vi "svfa_Locate Three Fingers (magnitude).vi"(2 "spectrum includes end points?":bool, 3 "criterion":T7={"Single/Multiple"=enum."Multiple Peaks", "Threshold"=0.0, "advanced search"={"approx freq. (optional)"=-1.0, "search (+/- % of Fsampl.)"=5.0}} {"advanced search"."search (+/- % of Fsampl.)" format="%0.2p"; "advanced search"."approx freq. (optional)" format="%0.2p"; "Threshold" format="%.2f"}, 4 "spectrum info":T1={"channel name"="", "description"="", "x-axis units"=0, "spectral info"={"spectrum type"=enum."Power [Magnitude^2]", "linear/dB"=enum."linear", "window"=0, "window size"=0, "FFT size"=0}, "engineering units"=0, "custom label"="", "dB reference [EU]"=0.0, "peak units"=enum."rms", "weighting filter"=0, "spectral density?"=FALSE, "unit label"="", "spectrum skewed?"=FALSE, "complimentary spectrum units"=enum."none"} {"x-axis units" items=["Time (s)"=0, "Frequency-CB (Hz)"=1, "Frequency-CPB (Hz)"=1248, "Frequency-Arbitrary (Hz)"=2357, "Quefrency (s)"=2, "Revolutions (rev)"=3, "Order"=4, "Speed (RPM)"=11, "Speed (rad/s)"=21, "Index"=65535]; "weighting filter" items=["Linear", "A-weighting", "B-weighting", "C-weighting", "ITU-R 468-4", "Dolby", "CCITT", "C-message", "Wb", "Wc", "Wd", "We", "Wf", "Wh", "Wj", "Wk", "Wm", "AES17 20 kHz lowpass", "AES17 40 kHz lowpass", "AES17 20 kHz highpass", "AES17 40 kHz highpass"]; "dB reference [EU]" format="%.2f"; "engineering units" items=["custom..."=0, "V"=1, "A"=21, "C"=30, "pC"=31, "s"=32, "-"=29, "Pa"=2, "N"=20, "g"=3, "m/s^2"=4, "m/s"=5, "m"=6, "mm/s"=12, "mm"=13, "micron/s"=14, "micron"=15, "in/s^2"=7, "in/s"=8, "in"=9, "mil/s"=10, "mil"=11, "rad/s^2"=16, "rad/s"=17, "rad"=18, "deg/s^2"=26, "deg/s"=27, "deg"=28, "RPM"=22, "cycle/s^2"=23, "Hz"=24, "cycle"=25, "strain"=19]; "spectral info"."window" items=["None "=0, "Hanning"=1, "Hamming"=2, "Blackman-Harris"=3, "Exact Blackman"=4, "Blackman"=5, "Flat Top"=6, "4 Term B-Harris "=7, "7 Term B-Harris"=8, "Low Sidelobe"=9, "Force - Exponential"=10, "Gaussian"=62]}, 5 "spectrum":cluster{"f0":dbl, "df":dbl, "magnitude":dbl[]} {"magnitude" format="%.2f"; "df" format="%.2f"; "f0" format="%.2f"}) -> (0 "number of tones":i32, 1 "three fingers (frequency normalized)":cluster{"f0":dbl, "df":dbl, "spectrum":dbl[]}[](array[cluster]) {"spectrum" format="%.2f"; "df" format="%.2e"; "f0" format="%.2e"})   [LabVIEW 2017]
uses:
  <vilib>/addons/_NISVFA/_Shared subVIs/Controls/svc_Spectrum Info.ctl
  <vilib>/addons/_NISVFA/_Shared subVIs/Controls/svc_X-Axis Units.ctl
  <vilib>/addons/_NISVFA/_Shared subVIs/Controls/svc_Spectrum Type.ctl
  <vilib>/addons/_NISVFA/_Shared subVIs/Controls/svc_Engineering Units Text Ring.ctl
  <vilib>/addons/_NISVFA/_Shared subVIs/Controls/svc_Weighting Filter Text Ring.ctl
  <vilib>/addons/_NISVFA/_Shared subVIs/Controls/svc_Complimentary Spectrum Units.ctl
  <vilib>/addons/_NISVFA/_Spectrum Processing/SVFA Get Spectrum Subset (1 Ch).vi
  <vilib>/addons/_NISVFA/_Shared subVIs/Common/svc_Spectrum Units.vi
  <vilib>/addons/_NISVFA/_Shared subVIs/Common/svc_Build Unit Label for Frequency Range.vi
  <vilib>/addons/_NISVFA/_Shared subVIs/Common/svc_Convert Frequency to Frequency String.vi
  <vilib>/addons/_NISVFA/_Shared subVIs/Common/svc_Caller VI Returned in Error Source.vi
  <vilib>/addons/_NISVFA/_Shared subVIs/Common/svc_Check Frequency Range in Spectrum.vi
  <vilib>/addons/_NISVFA/_Shared subVIs/Common/svc_Get Weighting Enum and Labels.vi
  <vilib>/addons/_NISVFA/_Shared subVIs/Common/svc_Unit Label Lexical Class.vi
  <vilib>/addons/_NISVFA/_Shared subVIs/Common/svc_Engineering Units to Unit Label.vi
  <vilib>/addons/_NISVFA/_Shared subVIs/Common/svc_Format Value (DBL).vi
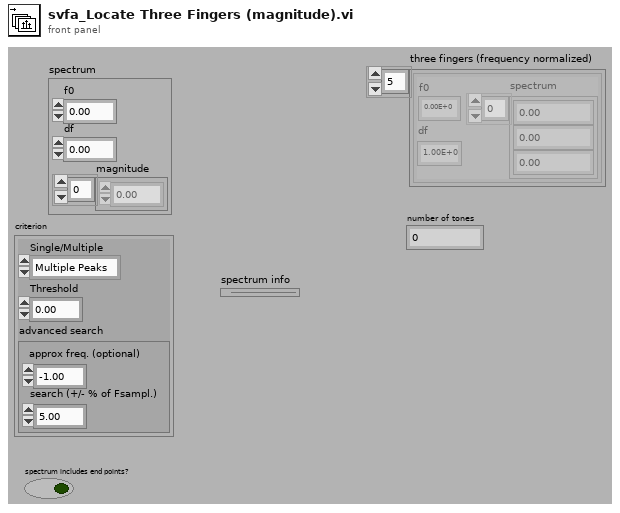
[diagram p1: front panel]
types:
  T1 = typedef "svc_Spectrum Info.ctl" = cluster{"channel name":string, "description":string, "x-axis units":T2, "spectral info":cluster{"spectrum type":T3, "linear/dB":enum16{"linear", "dB"}, "window":u16, "window size":i32, "FFT size":i32}, "engineering units":T4, "custom label":string, "dB reference [EU]":dbl, "peak units":enum16{"rms", "peak", "peak-peak"}, "weighting filter":T5, "spectral density?":bool, "unit label":string, "spectrum skewed?":bool, "complimentary spectrum units":T6}
  T2 = typedef "svc_X-Axis Units.ctl" = u16
  T3 = typedef "svc_Spectrum Type.ctl" = enum16{"FFT Spectrum [complex]", "Amplitude [Magnitude]", "Power [Magnitude^2]", "Cross Spectrum [complex]", "Frequency Response [Complex]"}
  T4 = typedef "svc_Engineering Units Text Ring.ctl" = u16
  T5 = typedef "svc_Weighting Filter Text Ring.ctl" = u16
  T6 = typedef "svc_Complimentary Spectrum Units.ctl" = enum16{"none", "radians", "degrees", "cycles", "imaginary"}
  T7 = cluster{"Single/Multiple":enum16{"Multiple Peaks", "Single Max Peak"}, "Threshold":dbl, "advanced search":cluster{"approx freq. (optional)":dbl, "search (+/- % of Fsampl.)":dbl}}
  T8 = cluster{"start frequency":dbl, "stop frequency":dbl}
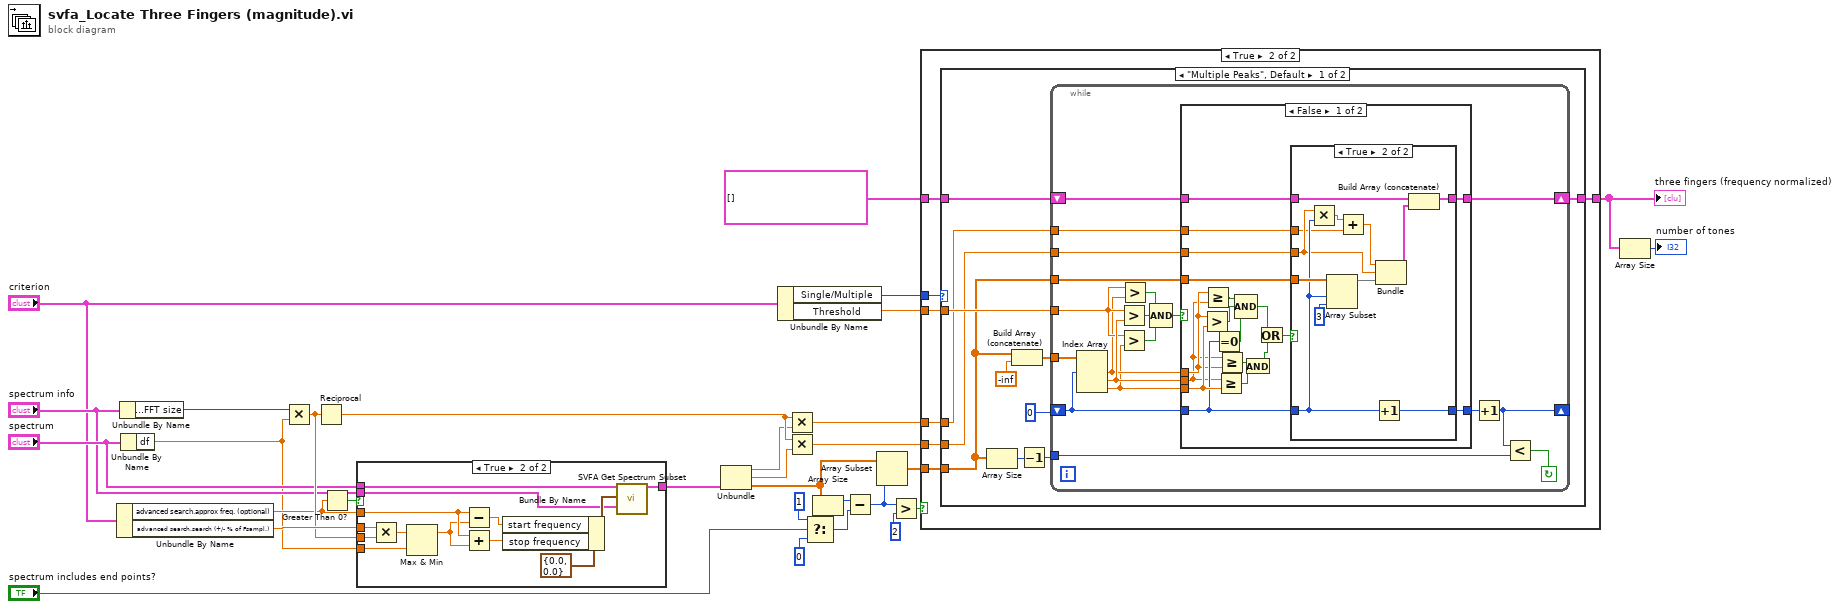
[diagram p0: block diagram]
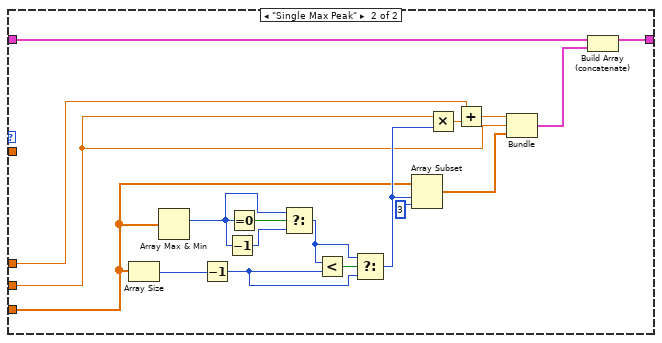
[diagram p6: hidden frame]
diagram:
  n1 = Unbundle By Name("criterion") -> ("advanced search.approx freq. (optional)"=w13:dbl, "advanced search.search (+/- % of Fsampl.)"=w15:dbl)
  n2 = Unbundle By Name("spectrum info") -> ("spectral info.FFT size"=w8:i32)
  n3 = Unbundle By Name("spectrum") -> ("df"=w4:dbl)
  n4 = Multiply(x=w8, y=w4) -> (x*y=w14:dbl)
  n5 = Reciprocal(x=w14) -> (1/x=w16:dbl)
  n6 = Greater Than 0?(x=w13) -> (x > 0?=w12:bool)
  n7 = case shown="True" w12 {
    tunnel: [w31 w34] -> w1
    tunnel: w15 -> [_ w43]
    tunnel: w14 -> [_ w42]
    tunnel: w13 -> [_ w41]
    tunnel: "spectrum" -> [w31 w39]
    tunnel: w4 -> [_ w37]
    tunnel: "spectrum info" -> [_ w33]
    frame False {
    }
    frame True {
      n8 = Multiply(x=w43, y=w42) -> (x*y=w36:dbl)
      n9 = Max & Min(x=w36, y=w37) -> (max(x,y)=w35:dbl)  [unwired: 1 out]
      n10 = Subtract(x=w41, y=w35) -> (x-y=w32:dbl)
      n11 = Add(x=w41, y=w35) -> (x+y=w40:dbl)
      n12 = Bundle By Name(cluster=T8 {"start frequency"=0.0, "stop frequency"=0.0} ("frequency range"), "start frequency"=w32, "stop frequency"=w40) -> (w38:T8)
      n13 = call-poly <vilib>:"SVFA Get Spectrum Subset.vi"("spectrum"=w39, "range"=w38, "spectrum info"=w33) -> ("spectrum subset"=w34:cluster{"x0":dbl, "dx":dbl, "magnitude":dbl[]})  [unwired: 11 in, 5 out]
    }
  }
  n14 = Unbundle(w1) -> ("x0"=w3:dbl, "dx"=w2:dbl, "magnitude"=w5:dbl[])
  n15 = Unbundle By Name("criterion") -> ("Single/Multiple"=w26:enum16{"Multiple Peaks", "Single Max Peak"}, "Threshold"=w27:dbl)
  n16 = Multiply(x=w16, y=w3) -> (x*y=w11:dbl)
  n17 = Multiply(x=w16, y=w2) -> (x*y=w10:dbl)
  n18 = Select(t=1, s="spectrum includes end points?", f=0) -> (s? t:f=w22:i32)
  n19 = Array Size(array=w5) -> (size(s)=w23:i32)
  n20 = Subtract(x=w23, y=w22) -> (x-y=w17:i32)
  n21 = Array Subset(array=w5, length=w17) -> (w18:dbl[])  [unwired: 1 in]
  n22 = Greater?(x=w17, y=2) -> (0:w29:bool)
  n23 = case shown="True" w29 {
    tunnel: w27 -> [_ w52]
    tunnel: w11 -> [_ w51]
    tunnel: w10 -> [_ w50]
    tunnel: [w45 w49] -> w25
    tunnel: w18 -> [_ w48]
    tunnel: cluster{"f0":dbl, "df":dbl, "spectrum":dbl[]}[] [] ("three fingers") -> [w45 w47]
    tunnel: w26 -> [_ w46]
    frame False {
    }
    frame True {
      n24 = case shown="\"Multiple Peaks\", Default" w46 {
        tunnel: w52 -> [w60 _]
        tunnel: w51 -> [w59 w124]
        tunnel: w50 -> [w58 w122]
        tunnel: [w57 w118] -> w49
        tunnel: w48 -> [w53 w117]
        tunnel: w47 -> [w54 w120]
        frame "Multiple Peaks", Default {
          n25 = Array Size(array=w53) -> (size(s)=w56:i32)
          n26 = Build Array (concatenate)(w53, -inf ("df")) -> (w62:dbl[])
          n27 = Decrement(x=w56) -> (x-1=w55:i32)
          n28 = while {
            tunnel: w55 -> [w71]
            tunnel: w58 -> [w75]
            tunnel: w59 -> [w76]
            tunnel: w53 -> [w77]
            shift-left: w54 -> [w78]
            shift-right: [w74] -> w57
            tunnel: w60 -> [w69]
            shift-left: 0 -> [w80]
            shift-right: [w72] -> _
            tunnel: w62 -> [w82]
            stop <- w73 continue-if-true
            n29 = Index Array(array=w82, index #1=w80) -> (element #1=w68:dbl, element #2=w70:dbl, element #3=w67:dbl)  [unwired: 2 in]
            n30 = Greater?(x=w69, y=w70) -> (0:w81:bool)
            n31 = Greater?(x=w69, y=w67) -> (0:w64:bool)
            n32 = Greater?(x=w69, y=w68) -> (0:w65:bool)
            n33 = Compound Arithmetic op=AND(w65, w81, w64) -> (w66:bool)
            n34 = case shown="False" w66 {
              tunnel: [w98 w116] -> w79
              tunnel: w80 -> [w88 w116]
              tunnel: w67 -> [w92 _]
              tunnel: w68 -> [w84 _]
              tunnel: w78 -> [w97 w115]
              tunnel: w77 -> [w96 _]
              tunnel: w76 -> [w95 _]
              tunnel: w75 -> [w94 _]
              tunnel: [w93 w115] -> w74
              tunnel: w70 -> [w83 _]
              frame False {
                n35 = Greater?(x=w84, y=w92) -> (0:w90:bool)
                n36 = Greater Or Equal?(x=w84, y=w83) -> (x >= y?=w91:bool)
                n37 = Equal To 0?(x=w88) -> (x = 0?=w89:bool)
                n38 = Greater Or Equal?(x=w83, y=w92) -> (x >= y?=w99:bool)
                n39 = Greater Or Equal?(x=w83, y=w84) -> (x >= y?=w100:bool)
                n40 = Compound Arithmetic op=AND(w91, w90, w89) -> (w85:bool)
                n41 = And(x=w100, y=w99) -> (x .and. y?=w87:bool)
                n42 = Or(x=w85, y=w87) -> (x .or. y?=w86:bool)
                n43 = case shown="True" w86 {
                  tunnel: w88 -> [w102 w112]
                  tunnel: [w102 w114] -> w98
                  tunnel: w97 -> [w101 w105]
                  tunnel: w96 -> [_ w113]
                  tunnel: w95 -> [_ w107]
                  tunnel: w94 -> [_ w109]
                  tunnel: [w101 w103] -> w93
                  frame False {
                  }
                  frame True {
                    n44 = Multiply(x=w109, y=w112) -> (x*y=w108:dbl)
                    n45 = Array Subset(array=w113, index=w112, length=3 ("Array Length")) -> (w110:dbl[])
                    n46 = Add(x=w108, y=w107) -> (x+y=w106:dbl)
                    n47 = Increment(x=w112) -> (x+1=w114:i32)
                    n48 = Bundle(w106, w109, w110) -> (w104:cluster{dbl, dbl, dbl[]})  [unwired: 1 in]
                    n49 = Build Array (concatenate)(w105, w104) -> (w103:cluster{"f0":dbl, "df":dbl, "spectrum":dbl[]}[])
                  }
                }
              }
              frame True {
              }
            }
            n50 = Increment(x=w79) -> (x+1=w72:i32)
            n51 = Less?(x=w72, y=w71) -> (x < y?=w73:bool)
          }
        }
        frame "Single Max Peak" {
          n52 = Array Size(array=w117) -> (size(s)=w126:i32)
          n53 = Array Max & Min(array=w117) -> (max index (indices)=w130:i32)  [unwired: 3 out]
          n54 = Decrement(x=w126) -> (x-1=w125:i32)
          n55 = Decrement(x=w130) -> (x-1=w131:i32)
          n56 = Equal To 0?(x=w130) -> (x = 0?=w132:bool)
          n57 = Select(t=w130, s=w132, f=w131) -> (s? t:f=w128:i32)
          n58 = Less?(x=w128, y=w125) -> (x < y?=w129:bool)
          n59 = Select(t=w128, s=w129, f=w125) -> (s? t:f=w127:i32)
          n60 = Array Subset(array=w117, index=w127, length=3 ("Array Length")) -> (w121:dbl[])
          n61 = Multiply(x=w122, y=w127) -> (x*y=w133:dbl)
          n62 = Add(x=w124, y=w133) -> (x+y=w123:dbl)
          n63 = Bundle(w123, w122, w121) -> (w119:cluster{dbl, dbl, dbl[]})  [unwired: 1 in]
          n64 = Build Array (concatenate)(w120, w119) -> (w118:cluster{"f0":dbl, "df":dbl, "spectrum":dbl[]}[])
        }
      }
    }
  }
  "three fingers (frequency normalized)" <- w25
  n65 = Array Size(array=w25) -> (size(s)=→"number of tones":i32)
